vi "Least Pth Norm Weighting Filter Design.vi"() -> ()   [LabVIEW 2023]
doc: "Demonstrates how to use the DFD Least Pth Norm Design VI to design advanced infinite impulse response (IIR) weighting filters. You can learn how to configure the controls to obtain the ideal frequency response of the filter you want to design.\n\nComplete the following steps to use this VI.\n1) Run the VI.\n2) Select one example filter in the <B>Examples</B> list. This VI provides pre-defined filter specifications for each example filter.\n3) View the <B>Specifications</B> page to study the corresponding settings that describe the ideal frequency response.\n4) Observe the magnitude response and the pole-zero plot to view the characteristics of the designed filter.\n5) Click the <B>STOP</B> button to stop this VI."
uses:
  <vilib>/addons/Digital Filter Design/_LpNorm.llb/dfd_Lp Norm Filter Type.ctl
  <vilib>/addons/Digital Filter Design/Design.llb/DFD Least Pth Norm Design by IRLS.vi
  <vilib>/addons/Digital Filter Design/NI_DigFilterLicensed.lvlib
panel:
  out "Status Info":string="Idle"
  out "Status LED":bool
  in  "Graph":enum32{"Magnitude Response", "Pole-Zero"}(tab)
  out "Magnitude Response":cluster{"Freqs":dbl[], dbl[]}[](graph)
  out "Z-Plane":T1(graph)
  in  "stop":bool
  in  "Selector":enum32{"Examples", "Specifications"}(tab)
  in  "Example List":i32(listbox)
  in  "Apply":bool
  in  "p":i32=128
  in  "Group Delay":dbl
  in  "Band Specifications":T2(array[cluster])=[{"frequency point"=[{"frequency"=0.0, "magnitude"=1.0, "weight"=1.0, "phase"=0.0}, {"frequency"=0.2, "magnitude"=1.0, "weight"=1.0, "phase"=0.0}]}, {"frequency point"=[{"frequency"=0.3, "magnitude"=0.0, "weight"=1.0, "phase"=0.0}, {"frequency"=0.5, "magnitude"=0.0, "weight"=1.0, "phase"=0.0}]}] {"frequency point"."weight" format="%.2f"}
  in  "Pole Radius Constraint":dbl=0.99 min=0.0
  in  "Sampling Frequency [Hz]":dbl=1.0 format="%.2f"
  in  "Order":cluster{"numerator":i32, "denominator":i32}={"numerator"=5, "denominator"=5}
  in  "Filter Type":T3
  # "Select Help>>Show Context Help and move the cursor over the VI icon for more information."
  # "freq"
  # "magnitude"
  # "weight"
  # "phase"
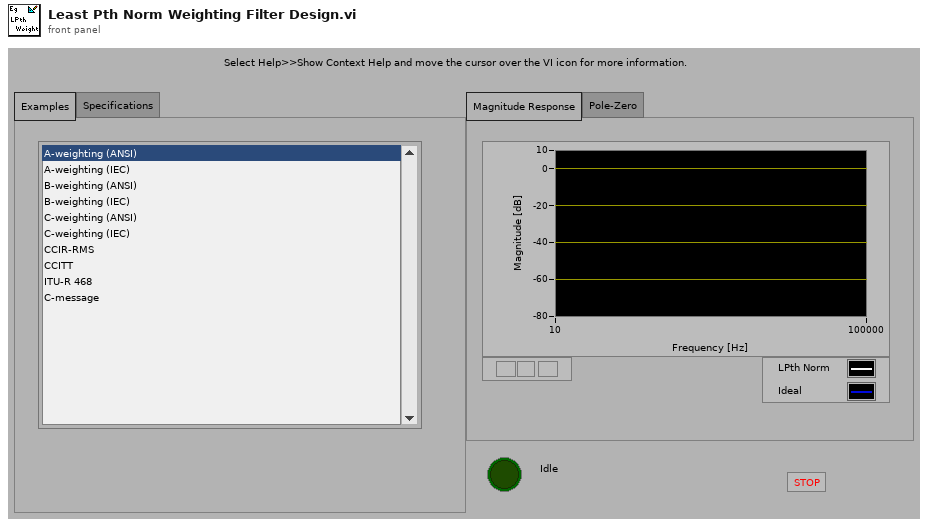
[diagram p1: front panel]
types:
  T1 = typedef "NI_DigFilterLicensed.lvlib/DFD Pole-Zero Plot.ctl" = cluster{dbl[], dbl[]}[]
  T2 = cluster{"frequency point":cluster{"frequency":dbl, "magnitude":dbl, "weight":dbl, "phase":dbl}[]}[]
  T3 = typedef "NI_DigFilterLicensed.lvlib/dfd_Lp Norm Filter Type.ctl" = enum16{"Symmetric", "Antisymmetric", "Differentiator", "Hilbert", "Minimum Phase", "Maximum Phase"}
  T4 = cluster{"pole radius constraint":dbl, "filter type":T3, "order":cluster{"num":i32, "den":i32}, "band specs":cluster{"frequency point":cluster{"frequency":dbl, "magnitude":dbl, "weight":dbl, "phase":dbl}[]}[], "group delay":dbl, "fs [Hz]":dbl, "p (128) 2":i32}
  T5 = typedef "NI_DigFilterLicensed.lvlib/DFD Filter Obj.ctl" = cluster{"mSRate_Fs":dbl, "mSRate_Version":string, "mSRate_Comments":string, "mSRate_OrgCoef":T6, "mSRate_CurCoef":T6, "mSRate_Quantized?":bool, "mSRate_QCoef":T6, "mSRate_QSettings":T8[], "mSRate_Order":i32, "mSRate_Scaling":cluster{"mSRate_ScaleByPowerOf2?":bool, "mSRate_ScaleType":T10}}
  T6 = typedef "NI_DigFilterLicensed.lvlib/DFD Filter Coef.ctl" = cluster{"type":T7, "gain":dbl, "coef a (k)":dbl[], "coef b (v)":dbl[]}
  T7 = typedef "NI_DigFilterLicensed.lvlib/DFD Filter Structure Type Selector.ctl" = enum16{"Undefined", "FIR Direct Form", "FIR Direct Form Transposed", "FIR Symmetric", "FIR Antisymmetric", "IIR Direct Form I", "IIR Direct Form I Transposed", "IIR Direct Form II", "IIR Direct Form II Transposed", "IIR Cascaded Second Order Sections Form I", "IIR Cascaded Second Order Sections Form I Transposed", "IIR Cascaded Second Order Sections Form II", "IIR Cascaded Second Order Sections Form II Transposed", "Lattice Allpass (basic sections)", "Lattice Allpass (one multiplier sections)", "Lattice Allpass (normalized sections)", "Lattice AR (basic sections)", "Lattice AR (one multiplier sections)", "Lattice AR (normalized sections)", "Lattice MA (minimum phase)", "Lattice MA (maximum phase)", "Lattice ARMA (basic sections)", "Lattice ARMA (one multiplier sections)", "Lattice ARMA (normalized sections)"}
  T8 = typedef "NI_DigFilterLicensed.lvlib/dfd_Internal Quantization Settings.ctl" = cluster{"source":T9, "wl":i16, "iwl":i16, "overflow mode":enum16{"Saturation", "Wrap"}, "rounding mode":enum16{"Nearest", "Truncation"}, "signed?":bool}
  T9 = typedef "NI_DigFilterLicensed.lvlib/dfd_Internal Quantization Srcs.ctl" = u16
  T10 = typedef "NI_DigFilterLicensed.lvlib/DFD Coef Norm Type.ctl" = enum16{"No Norm", "Time Domain 1-Norm", "Time Domain 2-Norm", "Time Domain Inf-Norm"}
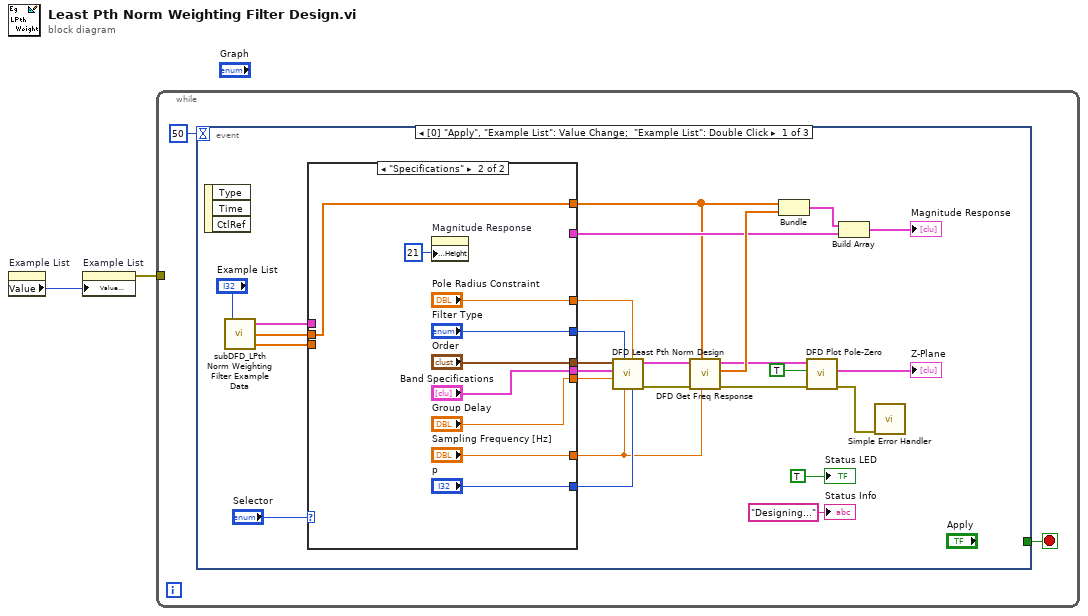
[diagram p0: block diagram]
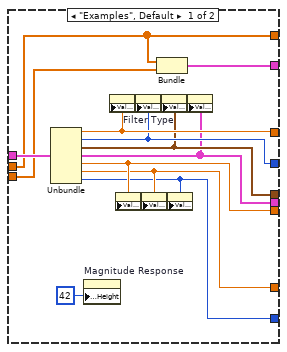
[diagram p2: hidden frame]
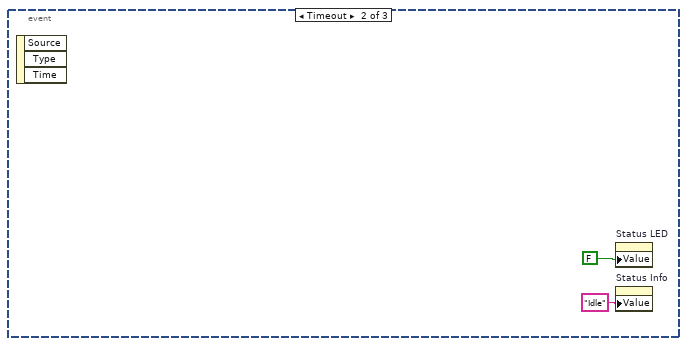
[diagram p3: hidden frame]
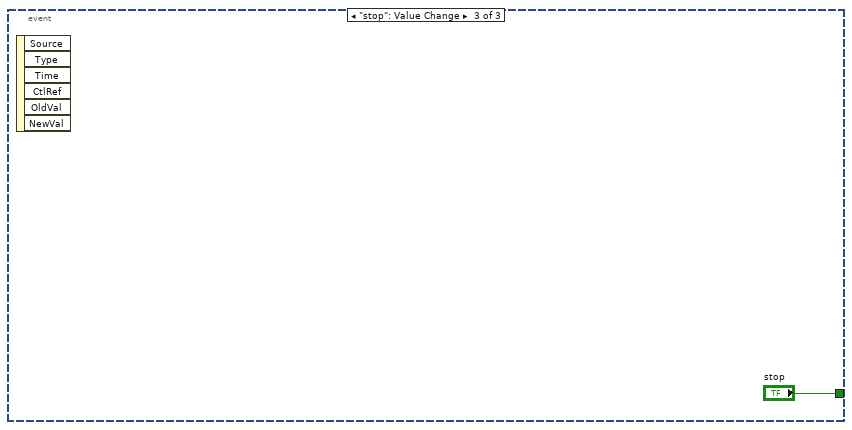
[diagram p4: hidden frame]
diagram:
  n1 = property on="Example List" class="LstBox (strict)"() -> ("Value"=w2:i32)  [unwired: 2 in, 2 out]
  n2 = property on="Example List" class="LstBox (strict)"("Value (Signaling)"=w2) -> (error out=w1:errorcluster)  [unwired: 2 in, 1 out]
  n3 = while {
    tunnel: w1 -> [_]
    stop <- w4 stop-if-true
    n4 = event shown="[0] \"Apply\", \"Example List\": Value Change;  \"Example List\": Double Click" {
      selector: _ -> [_ _ _]
      dyn-events: _ -> [_ _ _]
      timeout: 50 -> [_ _ _]
      tunnel: [_ _ "stop"] -> w4
      event "Apply", "Example List": Value Change; "Example List": Double Click {
        n5 = event-data() -> ()  [unwired: 4 out]
        n6 = call "subDFD_LPth Norm Weighting Filter Example Data.vi"("Example Idx"="Example List") -> ("Spec"=w12:T4, "Freqs"=w11:dbl[], "Ideal"=w10:dbl[])
        n7 = case shown="\"Specifications\"" "Selector" {
          tunnel: [w40 "Order"] -> w27
          tunnel: [w39 "Band Specifications"] -> w26
          tunnel: [w38 "Group Delay"] -> w25
          tunnel: [w37 "Sampling Frequency [Hz]"] -> w20
          tunnel: [w36 "p"] -> w24
          tunnel: [w41 "Filter Type"] -> w23
          tunnel: [w42 "Pole Radius Constraint"] -> w22
          tunnel: [w32 w51] -> w8
          tunnel: w12 -> [w35 _]
          tunnel: w11 -> [w32 w51]
          tunnel: w10 -> [w34 _]
          tunnel: [w33 _] -> w9
          frame "Examples", Default {
            n8 = Unbundle(w35) -> ("pole radius constraint"=w42:dbl, "filter type"=w41:T3, "order"=w40:cluster{"num":i32, "den":i32}, "band specs"=w39:T2, "group delay"=w38:dbl, "fs [Hz]"=w37:dbl, "p (128) 2"=w36:i32)
            n9 = property on="Magnitude Response" class="XYGraph (strict)"("Legend:Size:Height"=u32 42) -> ()  [unwired: 2 in, 2 out]
            n10 = property on="Pole Radius Constraint" class="DigNum (strict)"("Value"=w42) -> ()  [unwired: 2 in, 2 out]
            n11 = property on="Group Delay" class="DigNum (strict)"("Value"=w38) -> ()  [unwired: 2 in, 2 out]
            n12 = property on="Filter Type" class="Enum (strict)"("Value"=w41) -> ()  [unwired: 2 in, 2 out]
            n13 = property on="Sampling Frequency [Hz]" class="DigNum (strict)"("Value"=w37) -> ()  [unwired: 2 in, 2 out]
            n14 = Bundle("Freqs"=w32, "Ideal"=w34) -> (w33:cluster{"Freqs":dbl[], "Ideal":dbl[]})  [unwired: 1 out]
            n15 = property on="Order" class="Clust (strict)"("Value"=w40) -> ()  [unwired: 2 in, 2 out]
            n16 = property on="p" class="DigNum (strict)"("Value"=w36) -> ()  [unwired: 2 in, 2 out]
            n17 = property on="Band Specifications" class="Arr (strict)"("Value"=w39) -> ()  [unwired: 2 in, 2 out]
          }
          frame "Specifications" {
            n18 = property on="Magnitude Response" class="XYGraph (strict)"("Legend:Size:Height"=u32 21) -> ()  [unwired: 2 in, 2 out]
          }
        }
        n19 = call-poly <vilib>:"DFD Least Pth Norm Design.vi"("p (128)"=w24, "pole radius constraint"=w22, "fs [Hz]"=w20, "filter type"=w23, "group delay"=w25, "band specs"=w26, "order"=w27) -> ("error out"=w19:errorcluster, "filter out"=w21:T5)  [unwired: 1 in, 2 out]
        n20 = call <vilib>:"DFD Get Freq Response.vi"("fs [Hz]"=w20, "freq points [Hz]"=w8, "error in (no error)"=w19, "filter in"=w21) -> ("error out"=w15:errorcluster, "magnitude"=w18:dbl[], "filter out"=w16:T5)  [unwired: 3 in, 2 out]
        n21 = Bundle("Freqs"=w8, "magnitude"=w18) -> (w17:cluster{"Freqs":dbl[], "magnitude":dbl[]})  [unwired: 1 out]
        n22 = call <vilib>:"DFD Plot Pole-Zero.vi"("error in (no error)"=w15, "upper half plane only"=TRUE, "filter in"=w16) -> ("error out"=w28:errorcluster, "Z-Plane"=→"Z-Plane":T1)  [unwired: 7 out]
        n23 = Build Array(w17, w9) -> (→"Magnitude Response":cluster{"Freqs":dbl[], "Ideal":dbl[]}[])
        n24 = call <vilib>:"Simple Error Handler.vi"("error in (no error)"=w28) -> ()  [unwired: 1 in, 8 out]
        "Status LED" <- TRUE ("Status")
        "Status Info" <- "Designing..." ("String")
      }
      event Timeout {
        n25 = event-data() -> ()  [unwired: 4 out]
        n26 = property on="Status LED" class="Bool (strict)"("Value"=FALSE ("Status")) -> ()  [unwired: 2 in, 2 out]
        n27 = property on="Status Info" class="Str"("Value"="Idle" ("Status")) -> ()  [unwired: 2 in, 2 out]
      }
      event "stop": Value Change {
        n28 = event-data() -> ()  [unwired: 7 out]
      }
    }
  }
